vi "BlackjackProgramMarcoGonzalez.vi"() -> ()   [LabVIEW 2012]
doc: "This VI will allow the program to be a dealer and the user a player. The program includes:\n- a State Machine\n- total points visible to dealer and player\n- total # of cards visible to the dealer and player\n- Ace option available for the player\n- hit or stand option available for the player\n- status of win/lose or tie\n- directions on how to play blackjack game\n- key/legend on block diagram\n- name/period/date on front panel"
panel:
  out "Dealer Card 2":dbl
  out "Dealer Card 1":dbl
  out "User Card 2":dbl
  out "User Card 1":dbl
  out "Tie":bool
  out "Total # of Cards for Dealer":dbl
  out "Total # of Cards for User":dbl
  out "User Bust":bool
  out "Dealer Bust":bool
  out "User Wins":bool
  out "Dealer Wins":bool
  out "Total for Dealer":dbl
  out "Total for User":dbl
  # "Marco Gonzalez\nEA3  - 6th Period\n04 / 21 / 2017"
  # "Directions:\nThe user must select deal to start. They will select hit if they wish to gain more cards. If they wish to keep the cards dealt to them, then they must select stand.\nThe user may hit ace to either gain a card worth 1 or 11 points. The goal is to reach exactly 21 or be the closest to 21 once the game ends. The game can end\nif both the user and dealer hit stand or if either the user or dealer reahes exactly 21."
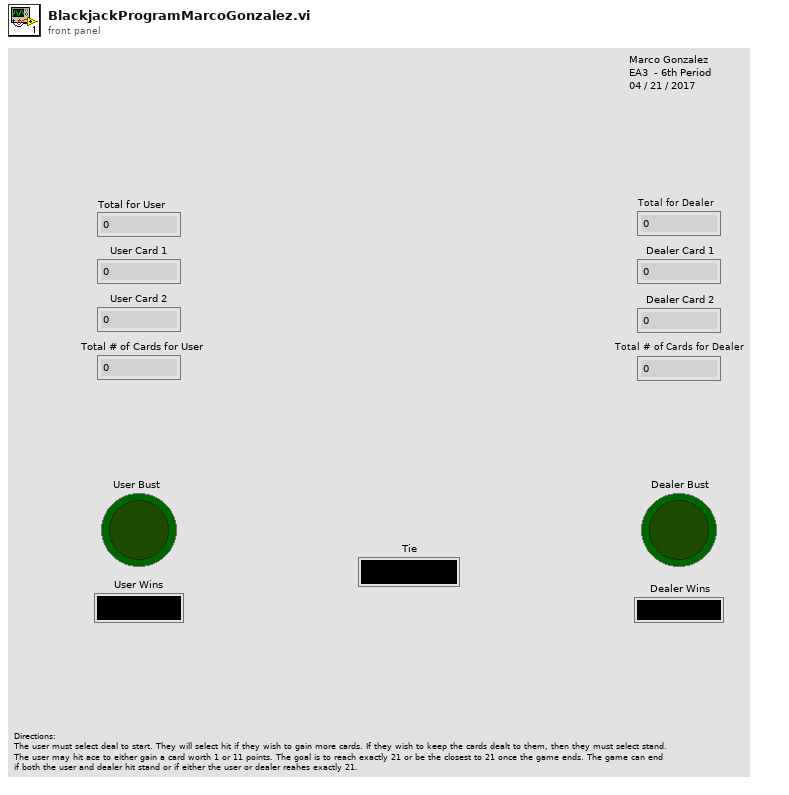
[diagram p1: front panel]
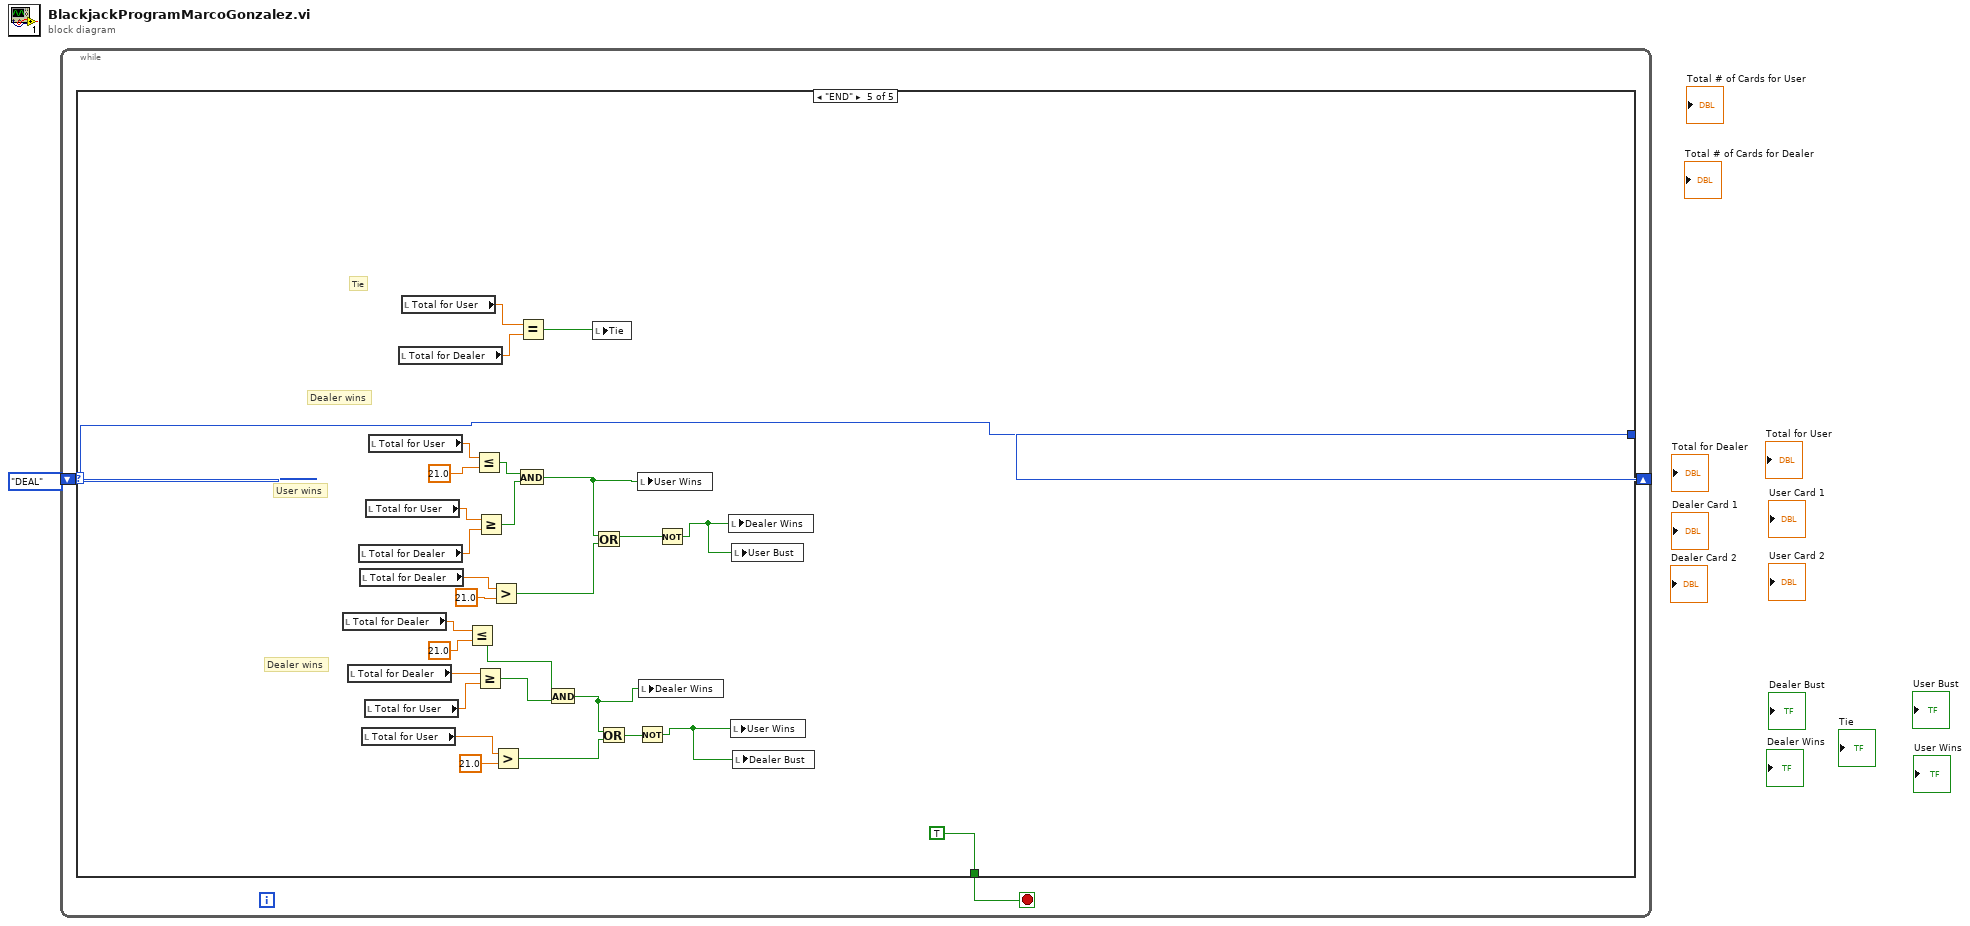
[diagram p0: block diagram]
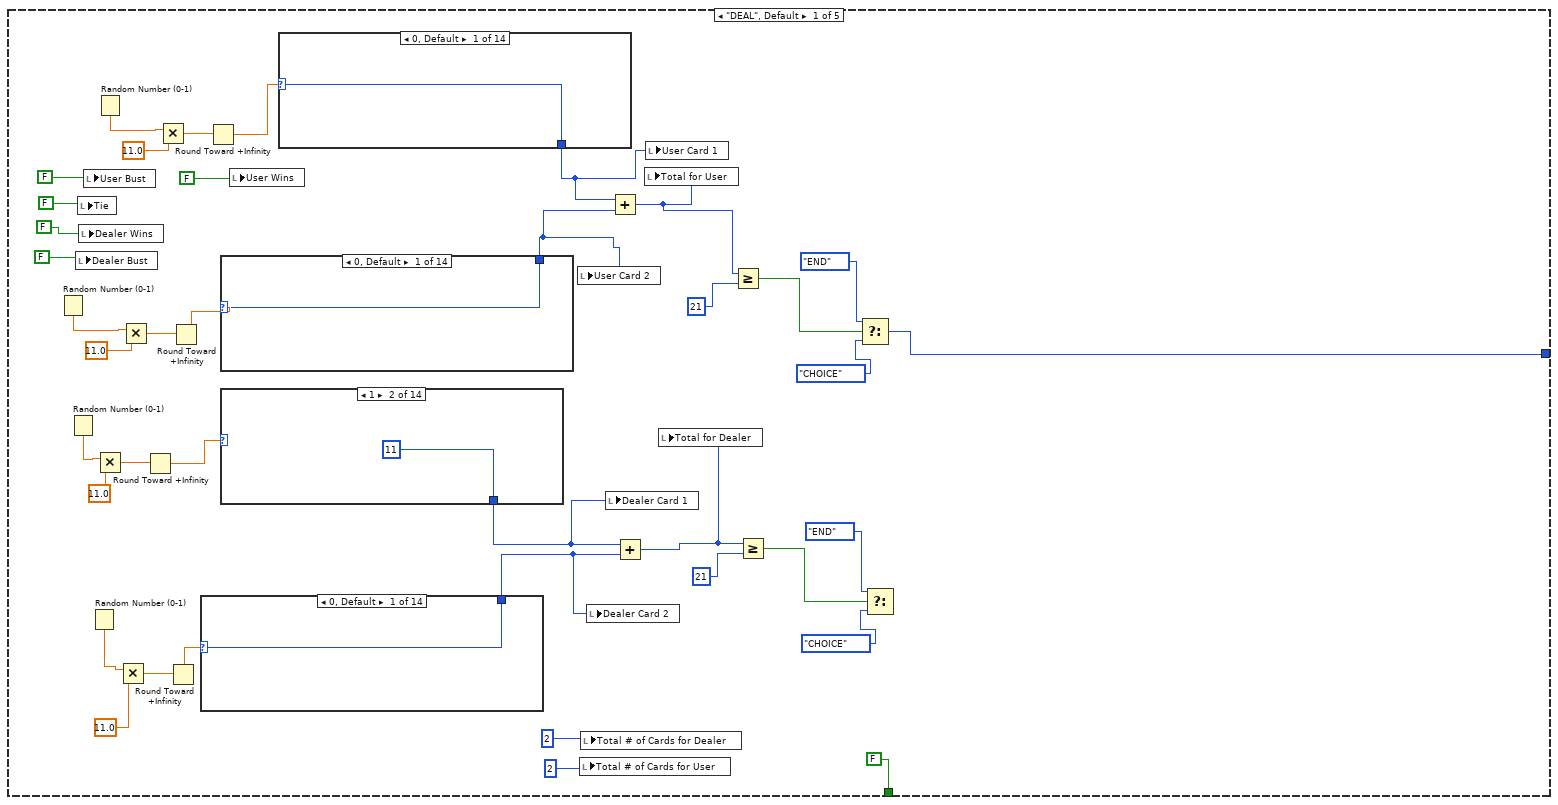
[diagram p2: hidden frame]
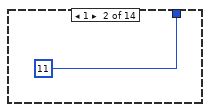
[diagram p3: hidden frame]
diagram:
  n1 = while {
    shift-right: [w2] -> _
    shift-left: enum16{"DEAL", "CHOICE", "HIT", "STAND", "END"}."DEAL" -> [w4]
    stop <- w3 stop-if-true
    n2 = case shown="\"END\"" w4 {
      selector: w4 -> [_ _ _ _ w171]
      tunnel: [FALSE FALSE FALSE FALSE TRUE] -> w3
      tunnel: [w32 w118 enum16{"DEAL", "CHOICE", "HIT", "STAND", "END"}."END" w151 w171] -> w2
      frame "DEAL", Default {
        n3 = Random Number (0-1)() -> (number: 0 to 1=w24:dbl)
        n4 = Random Number (0-1)() -> (number: 0 to 1=w19:dbl)
        n5 = local write "Dealer Bust"(FALSE) -> ()
        n6 = local write "Tie"(FALSE) -> ()
        n7 = local write "Dealer Wins"(FALSE) -> ()
        n8 = local write "User Bust"(FALSE) -> ()
        n9 = Random Number (0-1)() -> (number: 0 to 1=w15:dbl)
        n10 = Random Number (0-1)() -> (number: 0 to 1=w29:dbl)
        n11 = Multiply(x=w19, y=11.0) -> (x*y=w17:dbl)
        n12 = Multiply(x=w15, y=11.0) -> (x*y=w13:dbl)
        n13 = Multiply(x=w24, y=11.0) -> (x*y=w22:dbl)
        n14 = Round Toward +Infinity(x=w17) -> (ceil(x): smallest int >= x=w16:dbl)
        n15 = Multiply(x=w29, y=11.0) -> (x*y=w27:dbl)
        n16 = Round Toward +Infinity(x=w13) -> (ceil(x): smallest int >= x=w12:dbl)
        n17 = Round Toward +Infinity(x=w22) -> (ceil(x): smallest int >= x=w21:dbl)
        n18 = case shown="0, Default" w12 {
          selector: w12 -> [w44 _ w46 w47 w48 w49 w50 w51 w52 w53 w54 w55 w56 w57]
          tunnel: [w44 11 w46 w47 w48 w49 w50 w51 w52 w53 w54 w55 w56 w57] -> w10
          frame 0, Default {
          }
          frame 1 {
          }
          frame 2 {
          }
          frame 3 {
          }
          frame 4 {
          }
          frame 5 {
          }
          frame 6 {
          }
          frame 7 {
          }
          frame 8 {
          }
          frame 9 {
          }
          frame 10 {
          }
          frame 11 {
          }
          frame 12 {
          }
          frame 13 {
          }
        }
        n19 = Round Toward +Infinity(x=w27) -> (ceil(x): smallest int >= x=w26:dbl)
        n20 = case shown="0, Default" w21 {
          selector: w21 -> [w72 _ w80 w81 w82 w83 w84 w85 w86 w87 w88 w89 w90 w91]
          tunnel: [w72 w73 w80 w81 w82 w83 w84 w85 w86 w87 w88 w89 w90 w91] -> w20
          frame 0, Default {
          }
          frame 1 {
            n21 = Two Button Dialog(message="Choose: 1 or 11?", 1:"11" ("F button name (\"Cancel\")"), 2:"1" ("T button name (\"OK\")")) -> (T button?=w74:bool)
            n22 = case shown="False" w74 {
              tunnel: [11 1] -> w73
              frame False {
              }
              frame True {
              }
            }
          }
          frame 2 {
          }
          frame 3 {
          }
          frame 4 {
          }
          frame 5 {
          }
          frame 6 {
          }
          frame 7 {
          }
          frame 8 {
          }
          frame 9 {
          }
          frame 10 {
          }
          frame 11 {
          }
          frame 12 {
          }
          frame 13 {
          }
        }
        n23 = case shown="1" w16 {
          selector: w16 -> [w58 _ w60 w61 w62 w63 w64 w65 w66 w67 w68 w69 w70 w71]
          tunnel: [w58 11 w60 w61 w62 w63 w64 w65 w66 w67 w68 w69 w70 w71] -> w11
          frame 0, Default {
          }
          frame 1 {
          }
          frame 2 {
          }
          frame 3 {
          }
          frame 4 {
          }
          frame 5 {
          }
          frame 6 {
          }
          frame 7 {
          }
          frame 8 {
          }
          frame 9 {
          }
          frame 10 {
          }
          frame 11 {
          }
          frame 12 {
          }
          frame 13 {
          }
        }
        n24 = local write "User Wins"(FALSE) -> ()
        n25 = case shown="0, Default" w26 {
          selector: w26 -> [w92 _ w100 w101 w102 w103 w104 w105 w106 w107 w108 w109 w110 w111]
          tunnel: [w92 w93 w100 w101 w102 w103 w104 w105 w106 w107 w108 w109 w110 w111] -> w25
          frame 0, Default {
          }
          frame 1 {
            n26 = Two Button Dialog(message="Choose: 1 or 11?", 1:"11" ("F button name (\"Cancel\")"), 2:"1" ("T button name (\"OK\")")) -> (T button?=w94:bool)
            n27 = case shown="False" w94 {
              tunnel: [11 1] -> w93
              frame False {
              }
              frame True {
              }
            }
          }
          frame 2 {
          }
          frame 3 {
          }
          frame 4 {
          }
          frame 5 {
          }
          frame 6 {
          }
          frame 7 {
          }
          frame 8 {
          }
          frame 9 {
          }
          frame 10 {
          }
          frame 11 {
          }
          frame 12 {
          }
          frame 13 {
          }
        }
        n28 = local write "User Card 2"(w20) -> ()
        n29 = local write "Total # of Cards for User"(2) -> ()
        n30 = local write "Total # of Cards for Dealer"(2) -> ()
        n31 = local write "Dealer Card 2"(w10) -> ()
        n32 = local write "Dealer Card 1"(w11) -> ()
        n33 = Add(x=w25, y=w20) -> (x+y=w41:i32)
        n34 = Add(x=w11, y=w10) -> (x+y=w33:i32)
        n35 = local write "Total for User"(w41) -> ()
        n36 = local write "User Card 1"(w25) -> ()
        n37 = local write "Total for Dealer"(w33) -> ()
        n38 = Greater Or Equal?(x=w41, y=21) -> (x >= y?=w40:bool)
        n39 = Greater Or Equal?(x=w33, y=21) -> (x >= y?=w36:bool)
        n40 = Select(t=enum16{"DEAL", "CHOICE", "HIT", "STAND", "END"}."END", s=w40, f=enum16{"DEAL", "CHOICE", "HIT", "STAND", "END"}."CHOICE") -> (s? t:f=w32:enum16{"DEAL", "CHOICE", "HIT", "STAND", "END"})
        n41 = Select(t=enum16{"DEAL", "CHOICE", "HIT", "STAND", "END"}."END", s=w36, f=enum16{"DEAL", "CHOICE", "HIT", "STAND", "END"}."CHOICE") -> ()  [unwired: 1 out]
      }
      frame "HIT" {
        n42 = Random Number (0-1)() -> (number: 0 to 1=w127:dbl)
        n43 = local read "Total # of Cards for User"() -> (w115:dbl)
        n44 = Multiply(x=w127, y=11.0) -> (x*y=w125:dbl)
        n45 = Round Toward +Infinity(x=w125) -> (ceil(x): smallest int >= x=w113:dbl)
        n46 = case shown="0, Default" w113 {
          selector: w113 -> [w128 _ w136 w137 w138 w139 w140 w141 w142 w143 w144 w145 w146 w147]
          tunnel: [w128 w129 w136 w137 w138 w139 w140 w141 w142 w143 w144 w145 w146 w147] -> w112
          frame 0, Default {
          }
          frame 1 {
            n47 = Two Button Dialog(message="Choose: 1 or 11?", 1:"11" ("F button name (\"Cancel\")"), 2:"1" ("T button name (\"OK\")")) -> (T button?=w130:bool)
            n48 = case shown="False" w130 {
              tunnel: [11 1] -> w129
              frame False {
              }
              frame True {
              }
            }
          }
          frame 2 {
          }
          frame 3 {
          }
          frame 4 {
          }
          frame 5 {
          }
          frame 6 {
          }
          frame 7 {
          }
          frame 8 {
          }
          frame 9 {
          }
          frame 10 {
          }
          frame 11 {
          }
          frame 12 {
          }
          frame 13 {
          }
        }
        n49 = Add(x=1, y=w115) -> (x+y=w114:dbl)
        n50 = local write "Total # of Cards for User"(w114) -> ()
        n51 = local read "Total for User"() -> (w124:dbl)
        n52 = Add(x=w112, y=w124) -> (x+y=w119:dbl)
        n53 = Greater Or Equal?(x=w119, y=21) -> (x >= y?=w122:bool)
        n54 = local write "Total for User"(w119) -> ()
        n55 = local write "User Card 1"(w112) -> ()
        n56 = Select(t=enum16{"DEAL", "CHOICE", "HIT", "STAND", "END"}."END", s=w122, f=enum16{"DEAL", "CHOICE", "HIT", "STAND", "END"}."CHOICE") -> (s? t:f=w118:enum16{"DEAL", "CHOICE", "HIT", "STAND", "END"})
      }
      frame "STAND" {
      }
      frame "CHOICE" {
        n57 = Two Button Dialog(message="Do you wish to hit or stand?", 1:"STAND" ("F button name (\"Cancel\")"), 2:"HIT" ("T button name (\"OK\")")) -> (T button?=w154:bool)
        n58 = Select(t=enum16{"DEAL", "CHOICE", "HIT", "STAND"}."HIT", s=w154, f=enum16{"DEAL", "CHOICE", "HIT", "STAND"}."STAND") -> (s? t:f=w151:enum16{"DEAL", "CHOICE", "HIT", "STAND"})
      }
      frame "END" {
        # "Dealer wins"
        # "Tie"
        # "Dealer wins"
        # "User wins"
        n59 = local read "Total for Dealer"() -> (w178:dbl)
        n60 = local read "Total for Dealer"() -> (w176:dbl)
        n61 = local read "Total for Dealer"() -> (w180:dbl)
        n62 = local read "Total for Dealer"() -> (w168:dbl)
        n63 = local read "Total for User"() -> (w167:dbl)
        n64 = local read "Total for User"() -> (w175:dbl)
        n65 = local read "Total for User"() -> (w181:dbl)
        n66 = local read "Total for User"() -> (w184:dbl)
        n67 = local read "Total for Dealer"() -> (w185:dbl)
        n68 = local read "Total for User"() -> (w186:dbl)
        n69 = Less Or Equal?(x=w178, y=21.0) -> (x <= y?=w166:bool)
        n70 = Less Or Equal?(x=w184, y=21.0) -> (x <= y?=w182:bool)
        n71 = Greater Or Equal?(x=w176, y=w175) -> (x >= y?=w174:bool)
        n72 = Greater Or Equal?(x=w181, y=w180) -> (x >= y?=w179:bool)
        n73 = Greater?(x=w168, y=21.0) -> (0:w162:bool)
        n74 = Greater?(x=w167, y=21.0) -> (0:w165:bool)
        n75 = And(x=w182, y=w179) -> (x .and. y?=w161:bool)
        n76 = Equal?(x=w186, y=w185) -> (x = y?=w173:bool)
        n77 = And(x=w166, y=w174) -> (x .and. y?=w164:bool)
        n78 = local write "Tie"(w173) -> ()
        n79 = Or(x=w161, y=w162) -> (x .or. y?=w160:bool)
        n80 = Or(x=w164, y=w165) -> (x .or. y?=w163:bool)
        n81 = Not(x=w163) -> (.not. x?=w159:bool)
        n82 = local write "User Wins"(w161) -> ()
        n83 = local write "Dealer Wins"(w164) -> ()
        n84 = Not(x=w160) -> (.not. x?=w158:bool)
        n85 = local write "Dealer Wins"(w158) -> ()
        n86 = local write "User Wins"(w159) -> ()
        n87 = local write "User Bust"(w158) -> ()
        n88 = local write "Dealer Bust"(w159) -> ()
      }
    }
  }
